vi "Armed Configuration Response.vi"(8 "error in (no error)":errorcluster, 9 "Information":refnum<class "Information.lvclass">, 10 "Sender":string, 11 "Pulse Controller in":refnum<class "Pulse Controller.lvclass">) -> (0 "error out":errorcluster, 3 "Pulse Controller out":refnum<class "Pulse Controller.lvclass">)   [LabVIEW 2021, in "Pulse Controller.lvclass"]
uses:
  Pulse Controller.lvclass
  C:/Git/LabActor/Template Module/Template Module.lvclass
  Publish-Subscribe/Interfaces/Information/Information.lvclass
  NHMFL_Core/Libraries/Instruments/Results/Acquired Result/Acquired Result.lvclass
  Template Module/Template Module.lvclass/Template Module.ctl
  Template Module/Read Logger.vi
  Template Module/Write Logger.vi
  Measurements/Response Synchronizer/Response Synchronizer.lvclass
  Loggers/Logger/Logger.lvclass
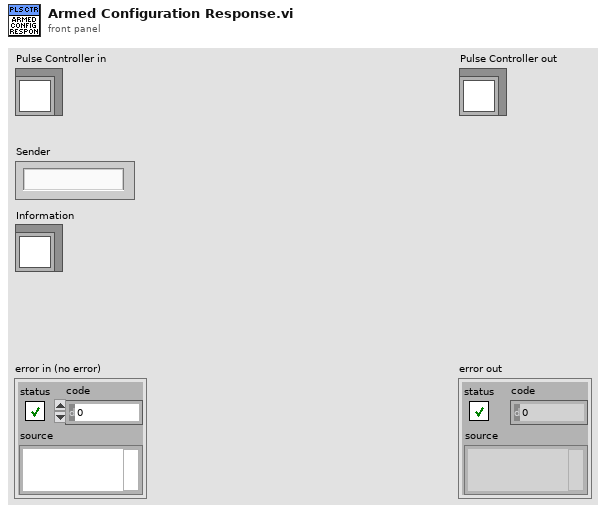
[diagram p1: front panel]
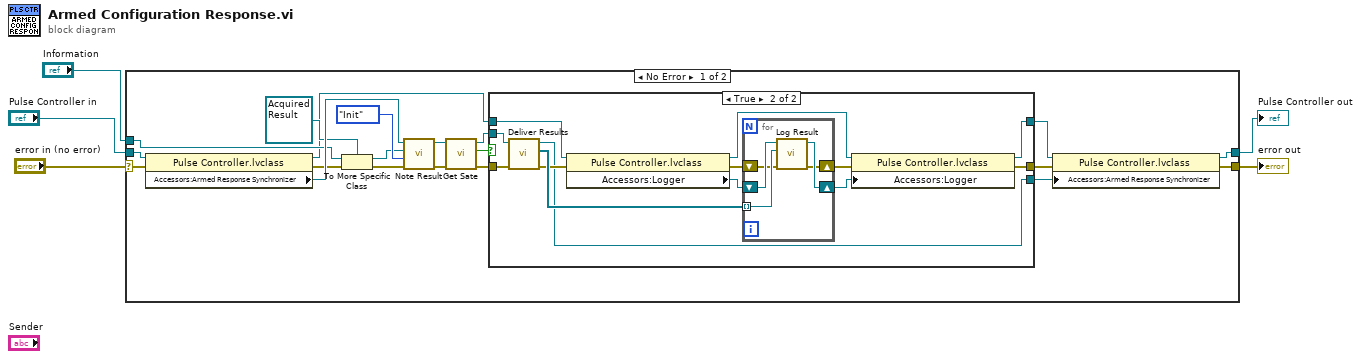
[diagram p0: block diagram]
diagram:
  n1 = case shown="No Error" "error in (no error)" {
    selector: "error in (no error)" -> [w18 w48]
    tunnel: [w7 w48] -> w4
    tunnel: [w9 w47] -> w2
    tunnel: "Pulse Controller in" -> [w25 w47]
    tunnel: "Information" -> [w22 _]
    frame No Error {
      n2 = property class="Pulse Controller.lvclass"(reference=w25, error in=w18) -> (reference out=w16:refnum<class "Pulse Controller.lvclass">, error out=w17:errorcluster, "Accessors:Armed Response Synchronizer"=w23:refnum<class "Response Synchronizer.lvclass">)
      n3 = To More Specific Class(target class=refnum<class "Acquired Result.lvclass"> refnum ("Acquired Result.lvclass"), reference=w22, error in=w17) -> (specific class reference=w19:refnum<class "Acquired Result.lvclass">, error out=w20:errorcluster)
      n4 = call-dynamic "Note Result.vi"("error in (no error)"=w20, "Stage"=enum16{"Init", "Work"}."Init", "Acquired Result.lvclass"=w19, "Response Synchronizer in"=w23) -> ("error out"=w14:errorcluster, "Response Synchronizer out"=w15:refnum<class "Response Synchronizer.lvclass">)  [unwired: 6 in]
      n5 = call-dynamic "Get Sate.vi"("error in (no error)"=w14, "Response Synchronizer in"=w15) -> ("error out"=w13:errorcluster, "Result ready"=w6:bool, "Response Synchronizer out"=w12:refnum<class "Response Synchronizer.lvclass">)  [unwired: 6 in, 1 out]
      n6 = case shown="True" w6 {
        tunnel: w13 -> [w28 w31]
        tunnel: w12 -> [w26 w33]
        tunnel: w16 -> [w27 w41]
        tunnel: [w28 w36] -> w8
        tunnel: [w27 w34] -> w11
        tunnel: [w26 w29] -> w10
        frame False {
        }
        frame True {
          n7 = call-dynamic "Deliver Results.vi"("error in (no error)"=w31, "Response Synchronizer in"=w33) -> ("error out"=w30:errorcluster, "Results"=w32:refnum<class "Acquired Result.lvclass">[], "Response Synchronizer out"=w29:refnum<class "Response Synchronizer.lvclass">)  [unwired: 7 in]
          n8 = property class="Pulse Controller.lvclass"(reference=w41, error in=w30) -> (reference out=w38:refnum<class "Pulse Controller.lvclass">, error out=w40:errorcluster, "Accessors:Logger"=w39:refnum<class "Logger.lvclass">)
          n9 = for {
            tunnel: w32 -> [w46] mode=indexing
            shift-right: [w44] -> w35
            shift-left: w39 -> [w45]
            shift-right: [w42] -> w37
            shift-left: w40 -> [w43]
            n10 = call-dynamic "Log Result.vi"("error in (no error)"=w43, "Result"=w46, "Logger in"=w45) -> ("error out"=w42:errorcluster, "Logger out"=w44:refnum<class "Logger.lvclass">)  [unwired: 7 in]
          }
          n11 = property class="Pulse Controller.lvclass"(reference=w38, error in=w37, "Accessors:Logger"=w35) -> (reference out=w34:refnum<class "Pulse Controller.lvclass">, error out=w36:errorcluster)
        }
      }
      n12 = property class="Pulse Controller.lvclass"(reference=w11, error in=w8, "Accessors:Armed Response Synchronizer"=w10) -> (reference out=w9:refnum<class "Pulse Controller.lvclass">, error out=w7:errorcluster)
    }
    frame Error {
    }
  }
  "error out" <- w4
  "Pulse Controller out" <- w2
